vi "user initialization.vi"(8 "error in":errorcluster, 10 "configuration in":refnum<class "control module configuration.lvclass">, 11 "fixed channel runtime in":refnum<class "ThreePhasePLL runtime.lvclass">) -> (0 "error out":errorcluster, 3 "fixed channel runtime out":refnum<class "ThreePhasePLL runtime.lvclass">)   [LabVIEW 2017, in "ThreePhasePLL runtime.lvclass"]
uses:
  ThreePhasePLL runtime.lvclass
  <vilib>/NI/DCAF/Tag Editor Core/control module/configuration/control module configuration.lvclass
  <vilib>/NI/DCAF/addons/InstructionFrameworkSupport/FPGA_FGV_action.ctl
  configuration/ThreePhasePLL configuration.lvclass
  <vilib>/userdefined/High Color/nirio_resource_hc.ctl
  configuration/ThreePhasePLL configuration.lvclass/ThreePhasePLL configuration.ctl
  ThreePhasePLL runtime.lvclass/ThreePhasePLL runtime.ctl
  <instrlib>/_niInstr/FIFO Register Bus/v1/Host/niInstr FIFO Register Bus v1 Host.lvclass
  C:/Program Files (x86)/National Instruments/LabVIEW 2017/instr.lib/_niInstr/Instruction Framework/v1/Host/Instruction Target/niInstr Instruction Target v1 Host.lvclass
  <vilib>/NI/PowerElectronicsControl/ThreePhasePLL/Interface/ThreePhasePLLInterface.lvlib
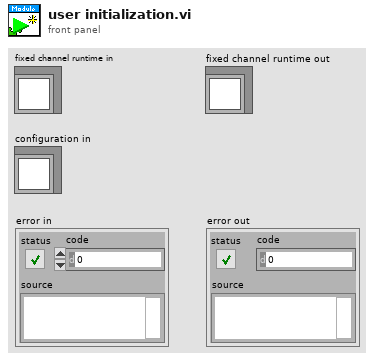
[diagram p1: front panel]
types:
  T1 = typedef "nirio_resource_hc.ctl" = tag
  T2 = typedef "FPGA_FGV_action.ctl" = enum16{"get FPGA", "set FPGA", "Close"}
  T3 = typedef "ThreePhasePLLInterface.lvlib/Configuration.ctl" = cluster{"PLLgains":T4, "PLLrange":T5, "dT":sgl, "expectedFreq":sgl, "lockDuration":sgl, "freqBoundaries":sgl, "adjustTheta":sgl, "HarmonicFilter":cluster{"enable":bool, "coeff":T6}}
  T4 = typedef "niFpgaPID_PIGains.ctl" = cluster{"proportional gain":sgl, "integral gain":sgl}
  T5 = typedef "niFpgaPID_OutputRange.ctl" = cluster{"output high (Inf)":sgl, "output low (-Inf)":sgl}
  T6 = typedef "ThreePhasePLL.lvlib/HarmonicFilter.ctl" = cluster{"ak":sgl, "bk":sgl}
  T7 = typedef "ThreePhasePLLInterface.lvlib/InterfaceRef.ctl" = cluster{"instruction target":refnum<class "niInstr Instruction Target v1 Host.lvclass">, "context":refnum<class "niInstr Instruction Framework Context v1 Host.lvclass">}
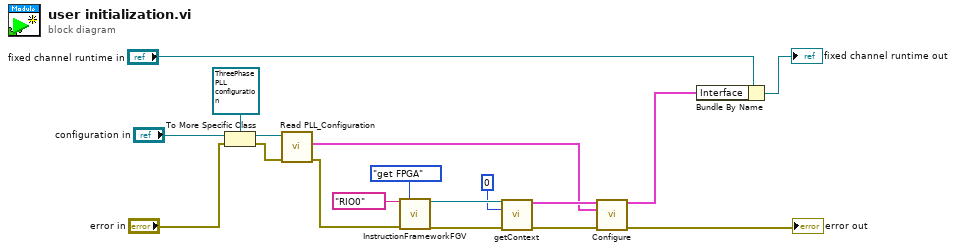
[diagram p0: block diagram]
diagram:
  n1 = To More Specific Class(target class=refnum<class "ThreePhasePLL configuration.lvclass"> refnum ("ThreePhasePLL configuration"), reference="configuration in", error in="error in") -> (specific class reference=w5:refnum<class "ThreePhasePLL configuration.lvclass">, error out=w3:errorcluster)
  n2 = call "Read PLL_Configuration.vi"("error in (no error)"=w3, "ThreePhasePLL configuration in"=w5) -> ("error out"=w8:errorcluster, "Configuration"=w2:T3)  [unwired: 7 in, 1 out]
  n3 = call <vilib>:"InstructionFrameworkFGV.vi"("RIO resource"=T1 "RIO0", "Action"=FPGA_FGV_action."get FPGA", "error in"=w8) -> ("session out"=w17:refnum<class "niInstr FIFO Register Bus v1 Host.lvclass">, "error out"=w15:errorcluster)  [unwired: 10 in, 1 out]
  n4 = call <vilib>:"getContext.vi"("instruction target in"=w17, "instance"=u8 0, "error in"=w15) -> ("Interface"=w11:T7, "error out"=w12:errorcluster)  [unwired: 11 in]
  n5 = call <vilib>:"Configure.vi"("Interface in"=w11, "Configuration"=w2, "error in"=w12) -> ("Interface out"=w10:T7, "error out"=→"error out":errorcluster)  [unwired: 11 in]
  n6 = Bundle By Name(cluster="fixed channel runtime in", "Interface"=w10) -> (→"fixed channel runtime out":refnum<class "ThreePhasePLL runtime.lvclass">)
